vi "GTRC HPOC UI.vi"() -> ()   [LabVIEW 2018]
uses:
  <vilib>/DAQmx/read.llb/DAQmx Read (Analog 1D DBL NChan 1Samp).vi
  <extravilib>/ChannelInstances/Lossy Stream-c(a[.](c(dbl,dbl,dbl,dbl)),stamp,a[.](dbl),c(dbl,dbl,dbl,dbl,dbl,dbl,dbl))/Read With Abort.vi
  <extravilib>/ChannelInstances/High Speed Stream-c(a[.](c(dbl,dbl,dbl,dbl)),stamp,a[.](dbl),c(dbl,dbl,dbl,dbl,dbl,dbl,dbl))/_Read For Replicate.vi
  <extravilib>/ChannelInstances/Lossy Stream-c(a[.](c(dbl,dbl,dbl,dbl)),stamp,a[.](dbl),c(dbl,dbl,dbl,dbl,dbl,dbl,dbl))/Write With Abort.vi
  <extravilib>/ChannelInstances/Lossy Stream-c(a[.](c(dbl,dbl,dbl,dbl)),stamp,a[.](dbl),c(dbl,dbl,dbl,dbl,dbl,dbl,dbl))/EndpointRead.vi
  <extravilib>/ChannelInstances/Lossy Stream-c(a[.](c(dbl,dbl,dbl,dbl)),stamp,a[.](dbl),c(dbl,dbl,dbl,dbl,dbl,dbl,dbl))/Endpoint.vi
  <extravilib>/ChannelInstances/Lossy Stream-c(a[.](c(dbl,dbl,dbl,dbl)),stamp,a[.](dbl),c(dbl,dbl,dbl,dbl,dbl,dbl,dbl))/Instantiate.vi
  <extravilib>/ChannelInstances/Lossy Stream-c(a[.](c(dbl,dbl,dbl,dbl)),stamp,a[.](dbl),c(dbl,dbl,dbl,dbl,dbl,dbl,dbl))/)Channel.vi
  <resource>/ChannelSupport/_ChannelSupport/WaitIfNeeded.vi
  <extravilib>/ChannelInstances/High Speed Stream-c(a[.](c(dbl,dbl,dbl,dbl)),stamp,a[.](dbl),c(dbl,dbl,dbl,dbl,dbl,dbl,dbl))/Instantiate.vi
  <extravilib>/ChannelInstances/High Speed Stream-c(a[.](c(dbl,dbl,dbl,dbl)),stamp,a[.](dbl),c(dbl,dbl,dbl,dbl,dbl,dbl,dbl))/)Channel.vi
  <extravilib>/ChannelInstances/High Speed Stream-c(a[.](c(dbl,dbl,dbl,dbl)),stamp,a[.](dbl),c(dbl,dbl,dbl,dbl,dbl,dbl,dbl))/Abort Signal/Init Signal.vi
  <vilib>/Utility/file.llb/Write Delimited Spreadsheet (string).vi
  <vilib>/DAQmx/create/channels.llb/DAQmx Create Channel (AI-Temperature-Thermocouple).vi
  <vilib>/DAQmx/configure/timing.llb/DAQmx Timing (Sample Clock).vi
  <vilib>/DAQmx/miscellaneous.llb/DAQmx Fill In Error Info.vi
  <extravilib>/ChannelInstances/High Speed Stream-c(a[.](c(dbl,dbl,dbl,dbl)),stamp,a[.](dbl),c(dbl,dbl,dbl,dbl,dbl,dbl,dbl)).lvlib
  <resource>/objmgr/daqmx.rc
  <extravilib>/ChannelInstances/Lossy Stream-c(a[.](c(dbl,dbl,dbl,dbl)),stamp,a[.](dbl),c(dbl,dbl,dbl,dbl,dbl,dbl,dbl)).lvlib
panel:
  out "Driving Variables":T1
  in  "Line Controls\n(Don't Delete)":T2(tab)
  in  "Line Flowrate Control":T3 {"Line 5" scale=0.0..5.0; "Line 4" scale=0.0..4.0; "Line 3" scale=0.0..3.0; "Line 2" scale=0.0..8.0; "Line 1" scale=0.0..9.0}
  in  "Temperatures Control":T3 {"Line 5" scale=0.0..10.0; "Line 4" scale=0.0..10.0; "Line 3" scale=0.0..10.0; "Line 2" scale=0.0..10.0; "Line 1" scale=0.0..10.0}
  in  "Pressure Controls":T3 {"Line 5" scale=0.0..10.0; "Line 4" scale=0.0..10.0; "Line 3" scale=0.0..10.0; "Line 2" scale=0.0..10.0; "Line 1" scale=0.0..10.0}
  in  "Species List":string[][](table)=[["Custom", "9999999999", ""], ["Methanol", "6.47", "19.93"], ["Butanol", "11.2", "33.075"], ["Propane", "15.67", "46.35"], ["Methane", "13.19", "50.00"], ["Hydrogen", "34.3", "119.96"], ["Ammonia", "6.0466", "22.5"], ["Pentane", "15.32", "45.36"], ["Butane", "14.98", "45.75"], ["Hexane", "15.24", "44.75"], ["Ethanol", "9", "26.70"], ["Empty (Not Used)", "0", "0"]]
  in  "Rig Temperature Tab Box\n(Don't Delete)":enum32{"Rig Temps Live", "Alarm Thresholds"}(tab)
  out "Rig Temperatures":T4
  in  "Rig Alarm Thresholds":T4
  out "DAQ Current Time":timestamp format="%<%X>T"
  in  "UI Refresh Rate (Hz)":u32=1 min=1 max=500 step=1
  out "Line Pressures":T5(graph)
  out "Line Temperatures":T5(graph)
  in  "Lines Tab Control\n(Don't delete)":enum32{"Live Data", "AFR Info", "Setup Lines"}(tab)
  out "Flowrate Data":T6(array[cluster]) {"Line Number" format="%#.1g"; "Temperature" format="%.2g"; "Pressure" format="%.2g"; "Flowrate" format="%.2g"}
  out "AFR Display":T7(array[cluster])
  in  "Line Setup":T8(array[cluster])
  out "Actual Sample Rate":dbl
  out "Export Timestamp":timestamp format="%<%H:%M:%S>T"
  out "UI Timestamp":timestamp format="%<%X\n%x>T"
  in  "file path (dialog if empty)":path
  out "Export Loop Status":T9(ring)
  in  "Start Recording?":bool
  in  "Stop Recording?":bool
  out "Acquisition Loop Status":T10(ring)
  in  "Begin Acquisition":bool
  in  "DAQ Properties":cluster{"Sample Rate [Hz]":dbl}={"Sample Rate [Hz]"=1.0} {"Sample Rate [Hz]" min=1.0 max=5000.0 step=1.0}
  # "Loop Status"
  # "Rig Temperatures [ °C]"
  # "Rig Thresholds [ °C]"
  # "Live \n Live Line Data"
  # "°C"
  # "Bar"
  # "g/s"
  # "Air-to-Fuel Ratios for each Line"
  # "Line Setup"
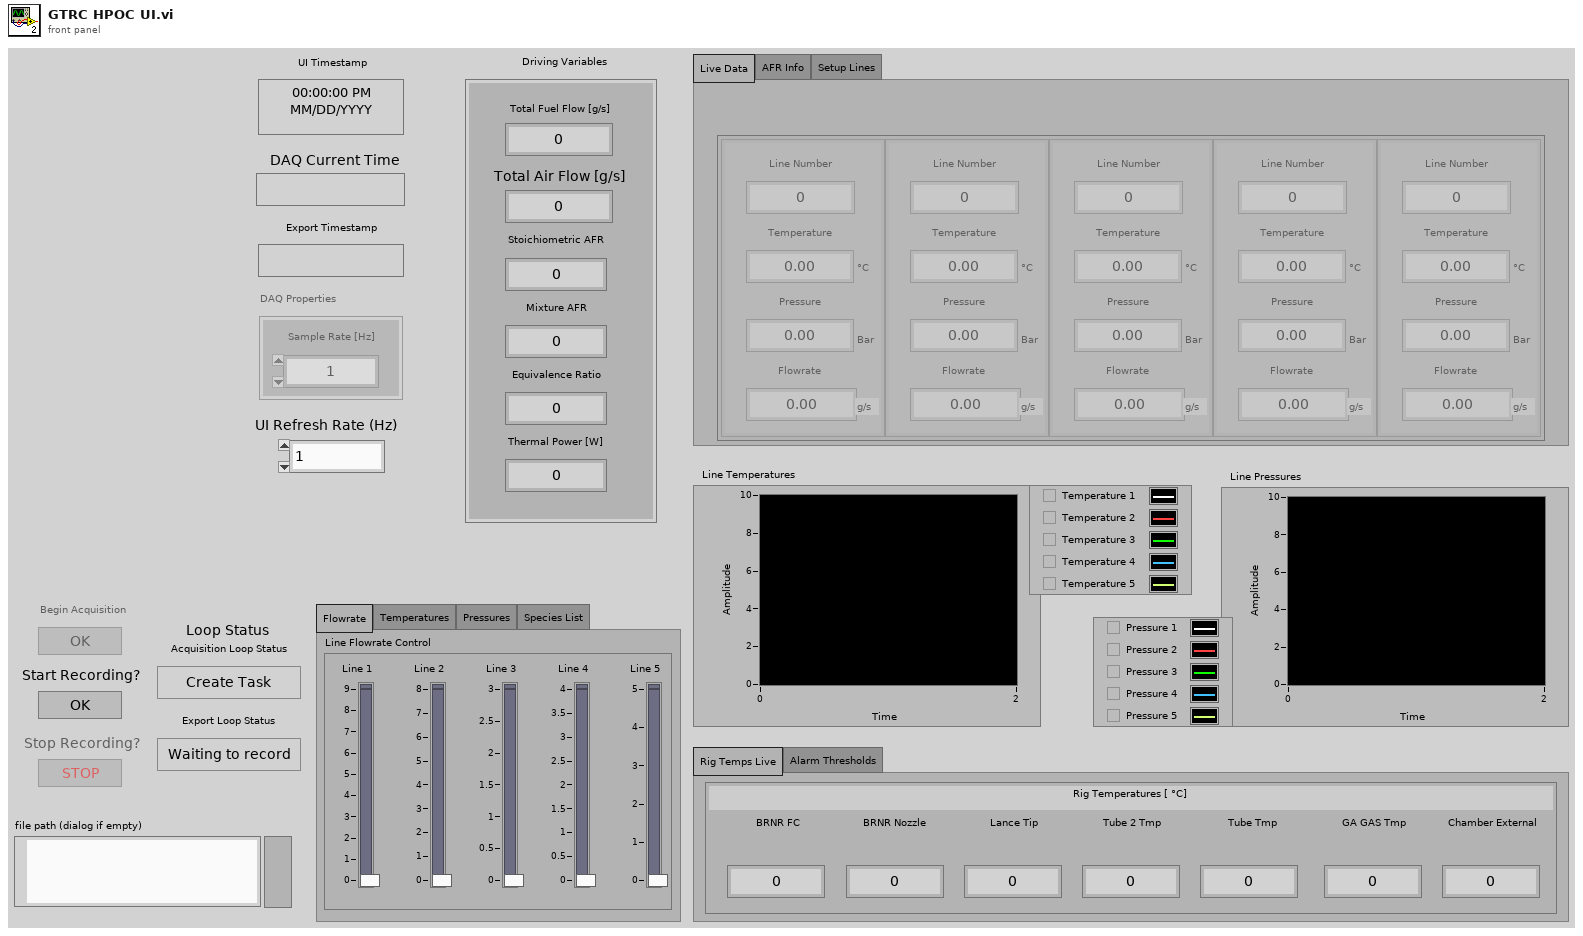
[diagram p1: front panel]
types:
  T1 = cluster{"Total Air Flow [g/s]":dbl, "Total Fuel Flow [g/s]":dbl, "Mixture AFR":dbl, "Stoichiometric AFR":dbl, "Equivalence Ratio":dbl, "Thermal Power [W]":dbl}
  T2 = enum32{"Flowrate", "Temperatures", "Pressures", "Species List"}
  T3 = cluster{"Line 1":dbl, "Line 2":dbl, "Line 3":dbl, "Line 4":dbl, "Line 5":dbl}
  T4 = cluster{"BRNR FC":dbl, "BRNR Nozzle":dbl, "Lance Tip":dbl, "Tube 2 Tmp":dbl, "Tube Tmp":dbl, "GA GAS Tmp":dbl, "Chamber External":dbl}
  T5 = cluster{"[0]":dbl, "[1]":dbl, "[2]":dbl, "[3]":dbl, "[4]":dbl}
  T6 = cluster{"Line Number":dbl, "Temperature":dbl, "Pressure":dbl, "Flowrate":dbl}[]
  T7 = cluster{"Line Number":i32, "AFR":dbl, "Species":enum16{"Empty (Not used)", "Custom", "Air", "Methanol", "Ethanol", "Butanol", "Propane", "Methane", "Hydrogen", "Pentane", "Butane", "Hexane"}}[]
  T8 = cluster{"Custom AFR":dbl, "Species":enum16{"Empty (Not used)", "Custom", "Air", "Methanol", "Ethanol", "Butanol", "Propane", "Methane", "Hydrogen", "Pentane", "Butane", "Hexane"}, "Custom Lower Heating Value [kJ/kg]":dbl}[]
  T9 = enum16{"Waiting to record", "Creating Spreadsheet", "Recording", "Finished Recording"}
  T10 = enum16{"Create Task", "Change Settings", "Check Settings", "Read Data", "End Task"}
  T11 = enum8{"Enabled", "Disabled", "Disabled and Grayed Out"}
  T12 = cluster{"Flowrate Data":cluster{"Line Number":dbl, "Temperature":dbl, "Pressure":dbl, "Flowrate":dbl}[], "Current Time":timestamp, "DAQmx Data":dbl[], "Rig Temperatures":cluster{"BRNR FC":dbl, "BRNR Nozzle":dbl, "Lance Tip":dbl, "Tube 2 Tmp":dbl, "Tube Tmp":dbl, "GA GAS Tmp":dbl, "Chamber External Temp":dbl}}
  T13 = cluster{"BRNR FC":dbl, "BRNR Nozzle":dbl, "Lance Tip":dbl, "Tube 2 Tmp":dbl, "Tube Tmp":dbl, "GA GAS Tmp":dbl, "Chamber External Temp":dbl}
  T14 = typedef "High Speed Stream-c(a[.](c(dbl,dbl,dbl,dbl)),stamp,a[.](dbl),c(dbl,dbl,dbl,dbl,dbl,dbl,dbl)).lvlib/)Channel.ctl" = refnum<queue>
  T15 = typedef "Lossy Stream-c(a[.](c(dbl,dbl,dbl,dbl)),stamp,a[.](dbl),c(dbl,dbl,dbl,dbl,dbl,dbl,dbl)).lvlib/)Channel.ctl" = refnum<queue>
  T16 = cluster{"Line":i32, "AFR":dbl, "Species":enum16{"Empty (Not used)", "Custom", "Air", "Methanol", "Ethanol", "Butanol", "Propane", "Methane", "Hydrogen", "Pentane", "Butane", "Hexane"}}
  T17 = enum16{"Empty (Not used)", "Custom", "Air", "Methanol", "Ethanol", "Butanol", "Propane", "Methane", "Hydrogen", "Pentane", "Butane", "Hexane"}
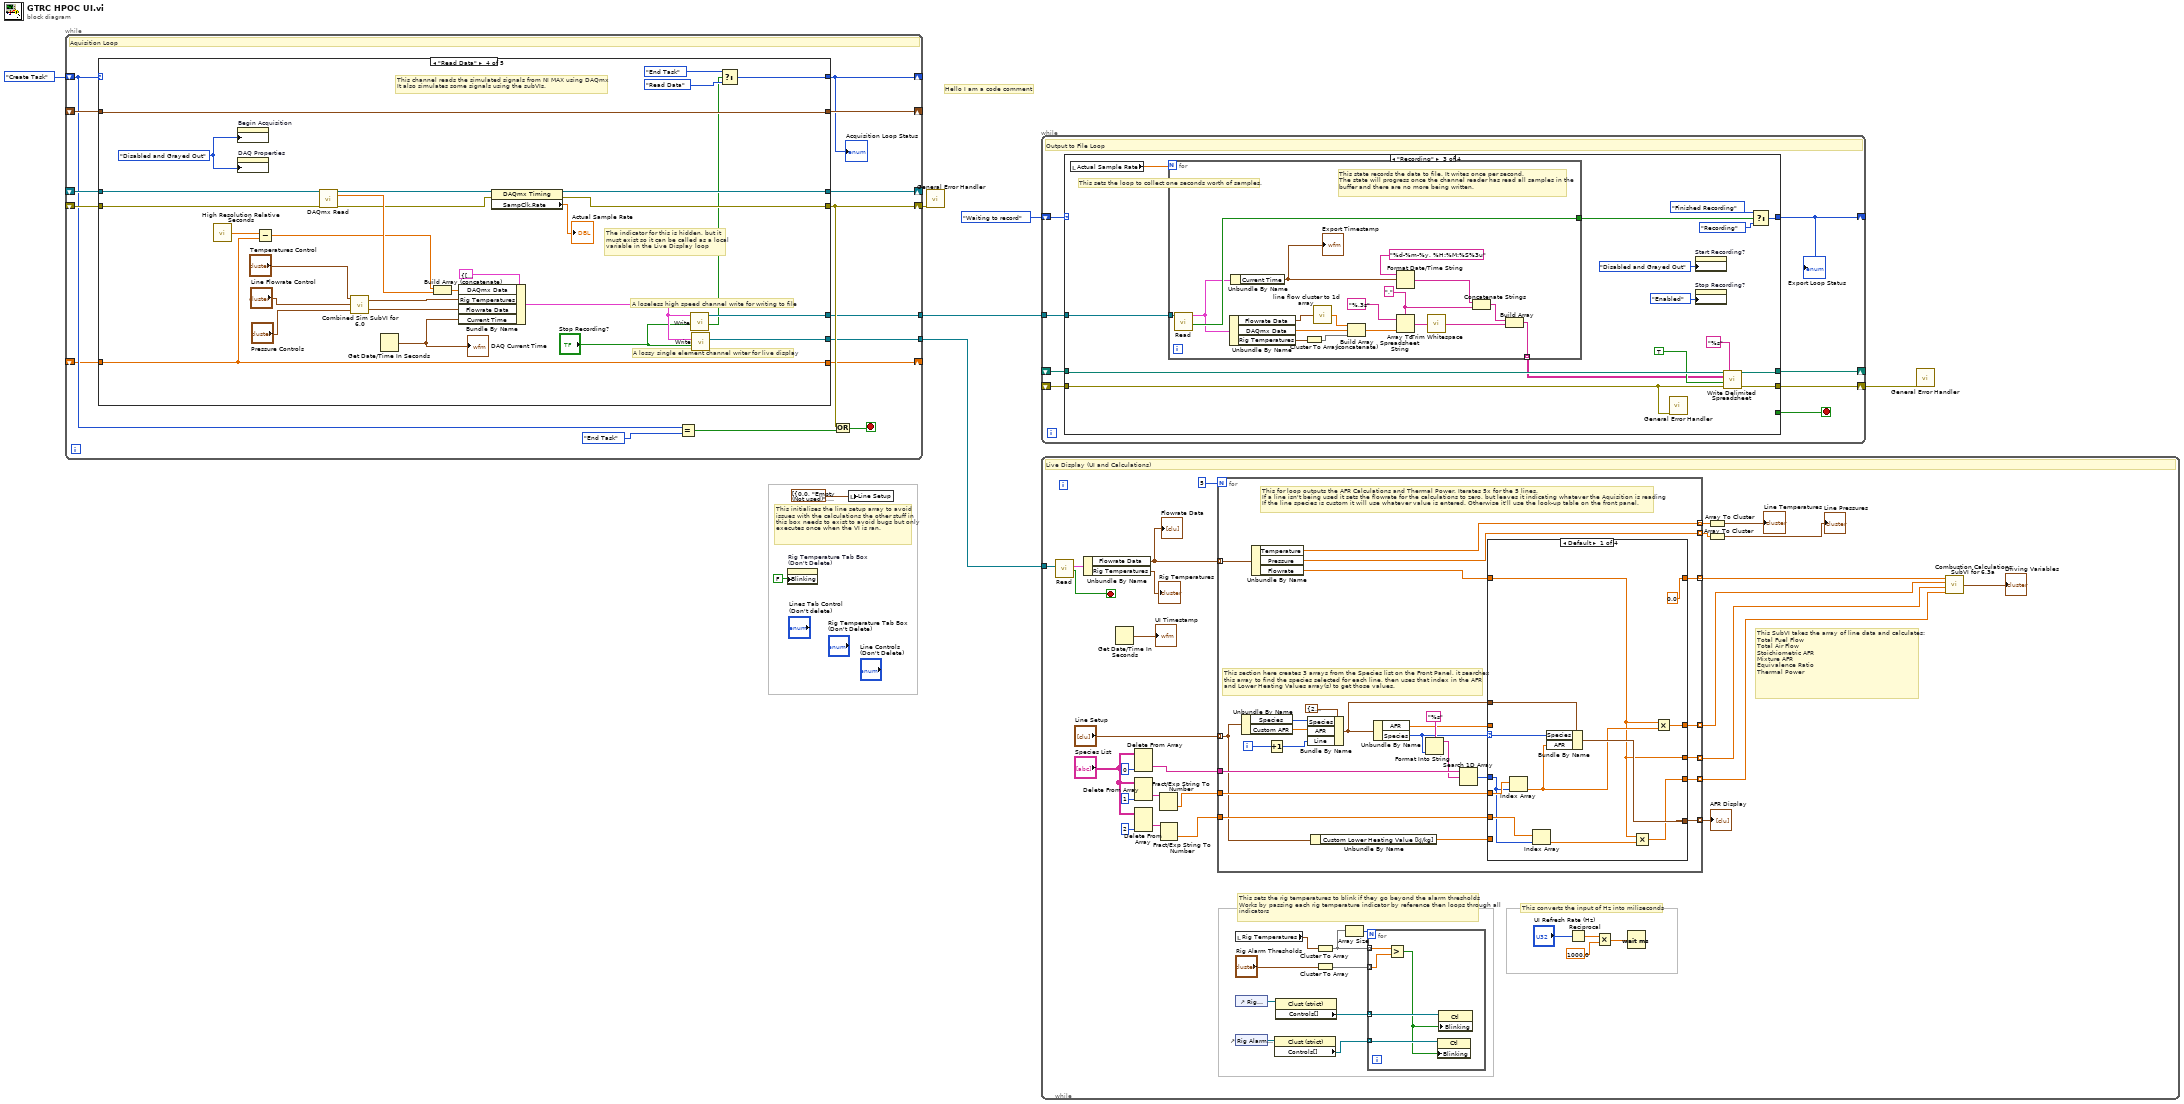
[diagram p0: block diagram]
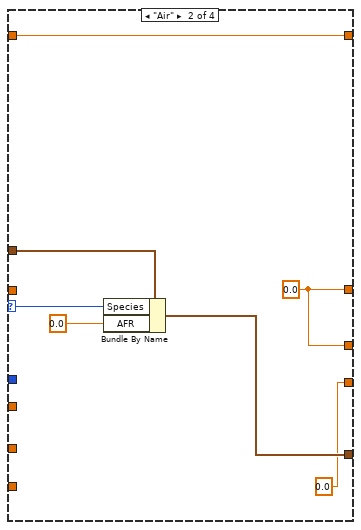
[diagram p2: hidden frame]
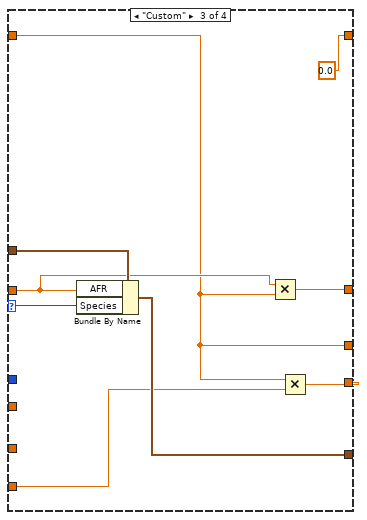
[diagram p3: hidden frame]
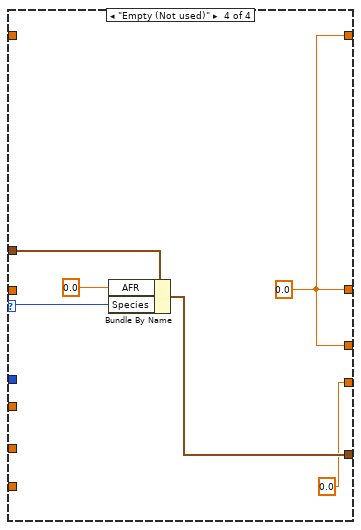
[diagram p4: hidden frame]
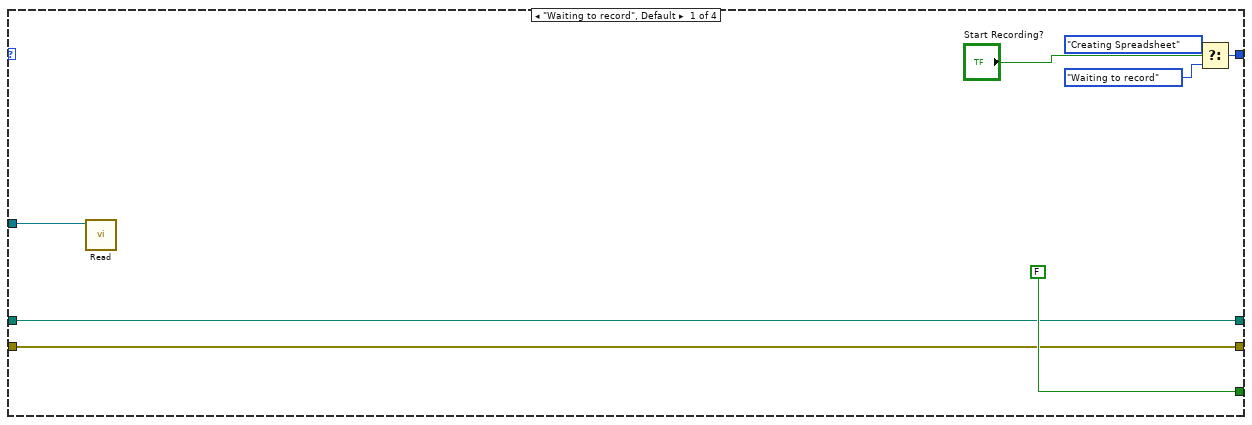
[diagram p5: hidden frame]
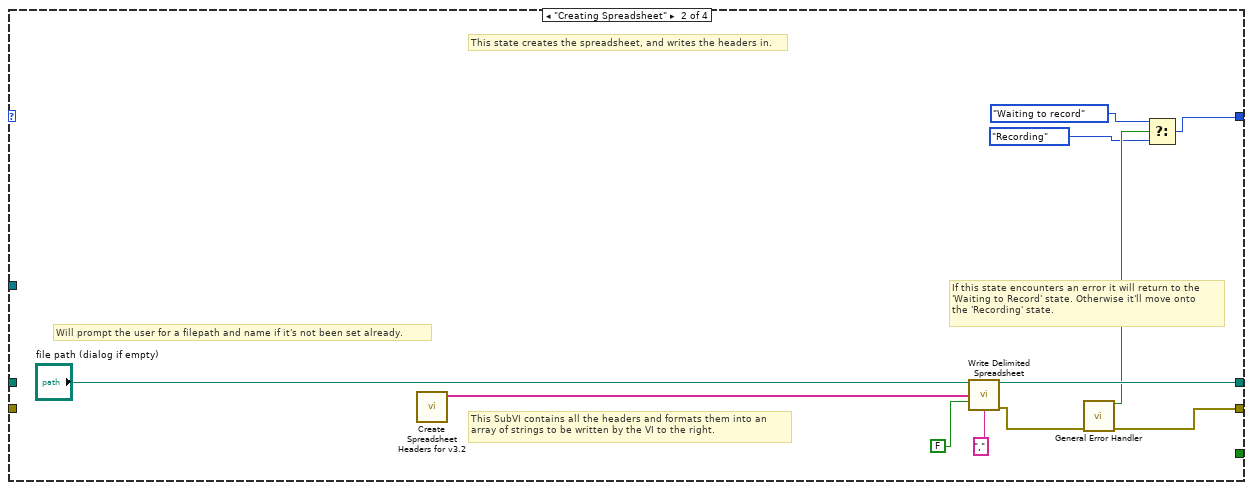
[diagram p6: hidden frame]
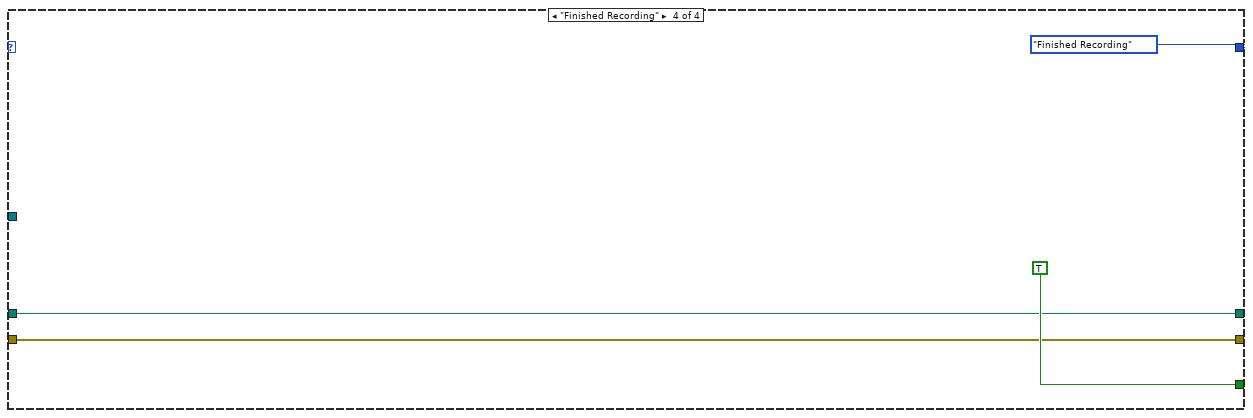
[diagram p7: hidden frame]
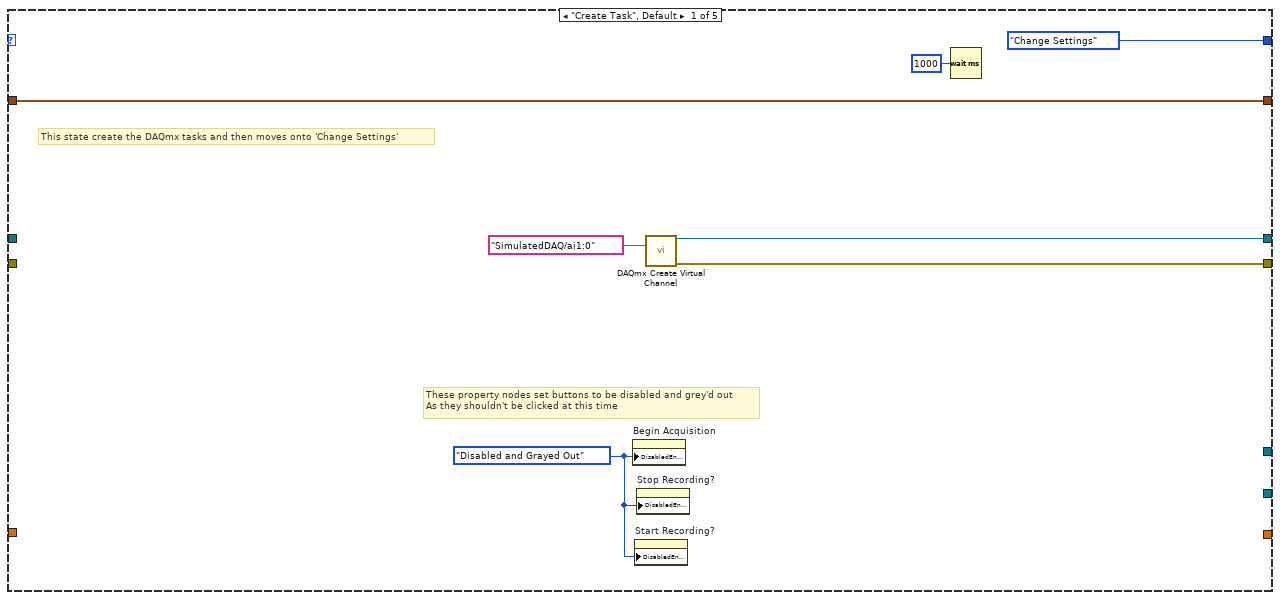
[diagram p8: hidden frame]
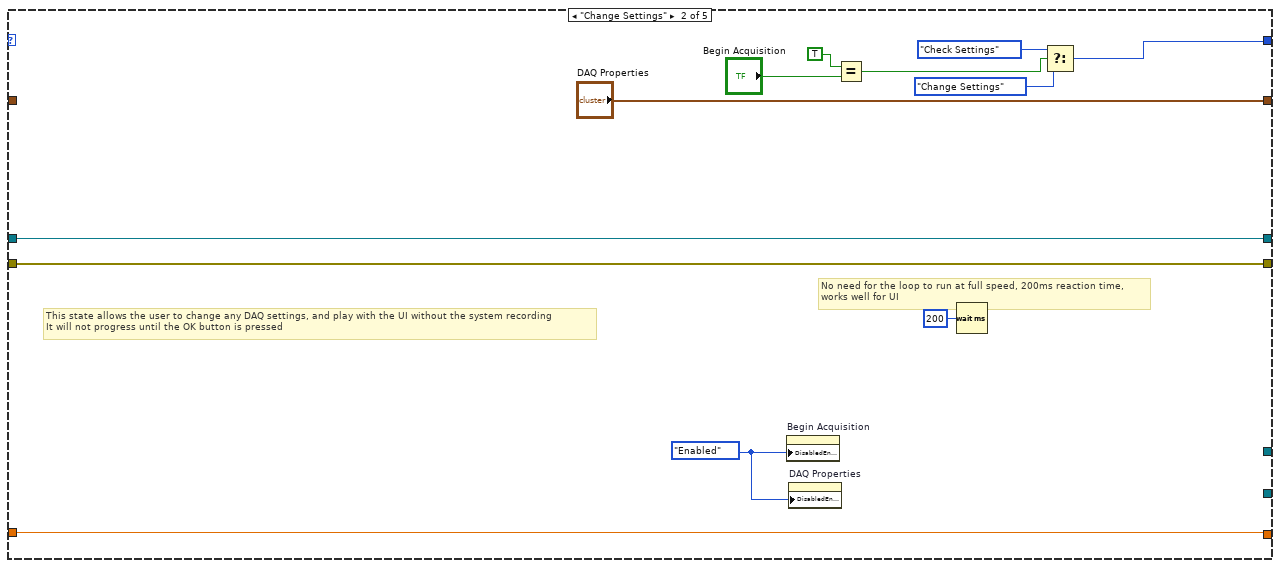
[diagram p9: hidden frame]
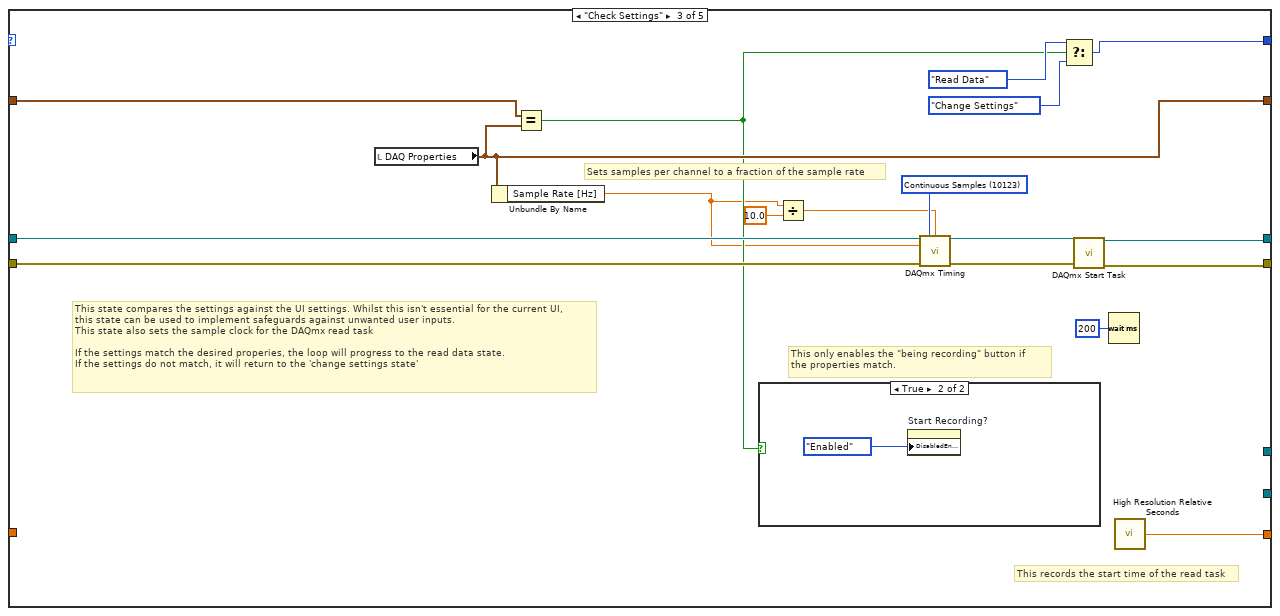
[diagram p10: hidden frame]
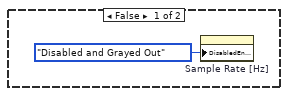
[diagram p11: hidden frame]
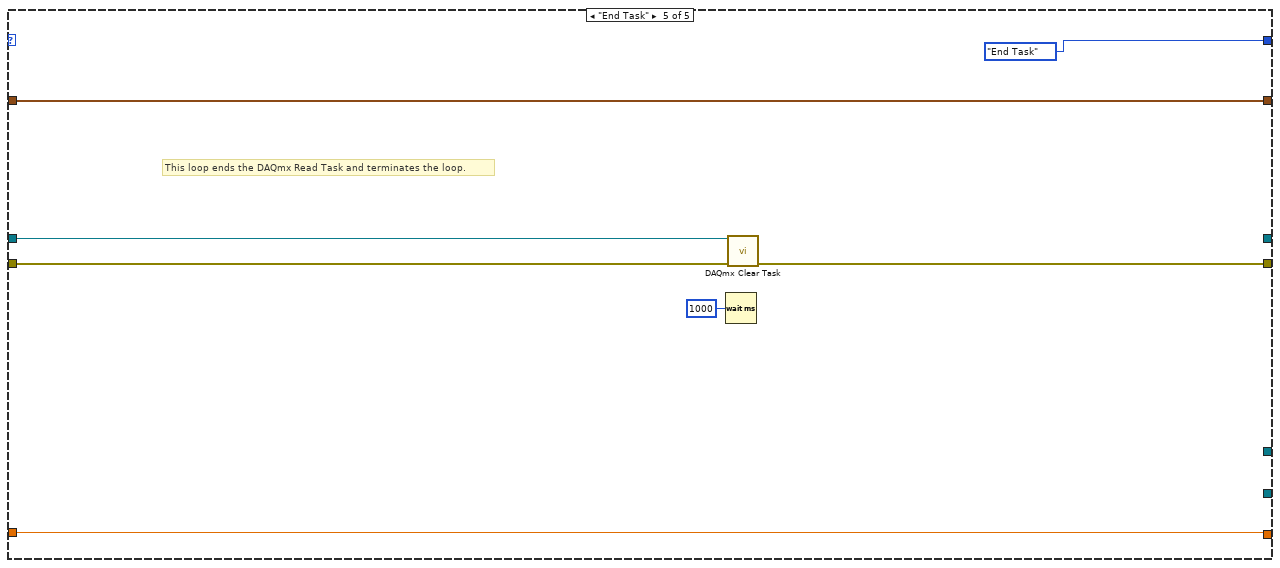
[diagram p12: hidden frame]
diagram:
  # "Hello I am a code comment"
  # "This initialises the line setup array to avoid issues with the calculations the other stuff in this box needs to exist to avoid bugs but only executes once when the VI is ran."
  n1 = while {
    shift-right: [w18] -> _
    shift-left: T10."Create Task" -> [w14]
    shift-right: [w23] -> _
    shift-left: _ -> [w21]
    shift-right: [w17] -> w4
    shift-left: _ -> [w20]
    shift-right: [w22] -> _
    shift-left: _ -> [w19]
    tunnel: [w13] -> w6
    tunnel: [w11] -> w3
    shift-right: [w9] -> _
    shift-left: _ -> [w10]
    stop <- w12 stop-if-true
    # "Aquisition Loop"
    n2 = case shown="\"Read Data\"" w14 {
      tunnel: [w30 w42 w50 w78 _] -> w23
      tunnel: [w29 w41 w49 w79 w98] -> w17
      tunnel: [T10."Change Settings" w35 w56 w87 T10."End Task"] -> w18
      tunnel: [w26 "DAQ Properties" w53 w89 w97] -> w22
      tunnel: w21 -> [_ w42 w55 w91 w95]
      tunnel: w20 -> [_ w41 w54 w90 w94]
      tunnel: w19 -> [w26 _ w60 w89 w97]
      tunnel: [_ _ _ w83 _] -> w13
      tunnel: [_ w31 w43 w74 w92] -> w9
      tunnel: w10 -> [_ w31 _ w74 w92]
      tunnel: [_ _ _ w71 _] -> w11
      frame "Create Task", Default {
        w24 = T11."Disabled and Grayed Out" ("Disabled")
        # "These property nodes set buttons to be disabled and grey'd out\nAs they shouldn't be clicked at this time"
        # "This state create the DAQmx tasks and then moves onto 'Change Settings'"
        n3 = property on="Begin Acquisition" class="Bool"("DisabledEnum"=w24) -> ()  [unwired: 2 in, 2 out]
        n4 = property on="Start Recording?" class="Bool"("DisabledEnum"=w24) -> ()  [unwired: 2 in, 2 out]
        n5 = property on="Stop Recording?" class="Bool"("DisabledEnum"=w24) -> ()  [unwired: 2 in, 2 out]
        n6 = call-poly <vilib>:"DAQmx Create Virtual Channel.vi"("physical channels"=tag "SimulatedDAQ/ai1:0") -> ("task out"=w30:refnum<k21>, "error out"=w29:errorcluster)  [unwired: 13 in]
        n7 = Wait (ms)(milliseconds to wait=u32 1000) -> ()  [unwired: 1 out]
      }
      frame "Change Settings" {
        w32 = T11."Enabled" ("Disabled")
        # "No need for the loop to run at full speed, 200ms reaction time,\nworks well for UI"
        # "This state allows the user to change any DAQ settings, and play with the UI without the system recording\nIt will not progress until the OK button is pressed"
        n8 = property on="Begin Acquisition" class="Bool"("DisabledEnum"=w32) -> ()  [unwired: 2 in, 2 out]
        n9 = property on="DAQ Properties" class="Clust (strict)"("DisabledEnum"=w32) -> ()  [unwired: 2 in, 2 out]
        n10 = Equal?(x=TRUE, y="Begin Acquisition") -> (x = y?=w37:bool)
        n11 = Wait (ms)(milliseconds to wait=u32 200) -> ()  [unwired: 1 out]
        n12 = Select(t=T10."Check Settings", s=w37, f=T10."Change Settings") -> (s? t:f=w35:T10)
      }
      frame "Check Settings" {
        w48 = 10123 items=["Finite Samples"=10178, "Continuous Samples"=10123, "Hardware Timed Single Point"=12522] ("sample mode")
        # "This records the start time of the read task"
        # "This only enables the \"being recording\" button if \nthe properties match."
        # "Sets samples per channel to a fraction of the sample rate"
        # "This state compares the settings against the UI settings. Whilst this isn't essential for the current UI, \nthis state can be used to implement safeguards against unwanted user inputs.\nThis state also sets the sample clock for the DAQmx read task\n\nIf the settings match the desired properies, the loop will progress to the read data state.\nIf the settings do not match, it will return to the 'change settings state'"
        n13 = local read "DAQ Properties"() -> (w53:cluster{"Sample Rate [Hz]":dbl})
        n14 = Unbundle By Name(w53) -> ("Sample Rate [Hz]"=w45:dbl)
        n15 = Equal?(x=w60, y=w53) -> (x = y?=w47:bool)
        n16 = case shown="True" w47 {
          frame False {
            n17 = property on="Sample Rate [Hz]" class="DigNum (strict)"("DisabledEnum"=T11."Disabled and Grayed Out" ("Disabled")) -> ()  [unwired: 2 in, 2 out]
          }
          frame True {
            n18 = property on="Start Recording?" class="Bool"("DisabledEnum"=T11."Enabled" ("Disabled")) -> ()  [unwired: 2 in, 2 out]
          }
        }
        n19 = Divide(x=w45, y=10.0) -> (x/y=w44:dbl)
        n20 = call-poly <vilib>:"DAQmx Timing.vi"("task/channels in"=w55, "sample mode"=w48, "samples per channel"=w44, "rate"=w45, "error in"=w54) -> ("task out"=w52:refnum<k21>, "error out"=w51:errorcluster)  [unwired: 9 in]
        n21 = Select(t=T10."Read Data", s=w47, f=T10."Change Settings") -> (s? t:f=w56:T10)
        n22 = call <vilib>:"DAQmx Start Task.vi"("task/channels in"=w52, "error in"=w51) -> ("task out"=w50:refnum<k21>, "error out"=w49:errorcluster)  [unwired: 12 in]
        n23 = Wait (ms)(milliseconds to wait=u32 200) -> ()  [unwired: 1 out]
        n24 = call <vilib>:"High Resolution Relative Seconds.vi"() -> ("relative seconds"=w43:dbl)
      }
      frame "Read Data" {
        w82 = T11."Disabled and Grayed Out" ("Disabled")
        # "This channel reads the simulated signals from NI MAX using DAQmx\nIt also simulates some signals using the subVIs."
        # "A lossy single element channel writer for live display"
        # "A loseless high speed channel write for writing to file"
        # "The indicator for this is hidden, but it\nmust exist so it can be called as a local \nvariable in the Live Display loop"
        n25 = call <vilib>:"High Resolution Relative Seconds.vi"() -> ("relative seconds"=w76:dbl)
        n26 = property on="Begin Acquisition" class="Bool"("DisabledEnum"=w82) -> ()  [unwired: 2 in, 2 out]
        n27 = property on="DAQ Properties" class="Clust (strict)"("DisabledEnum"=w82) -> ()  [unwired: 2 in, 2 out]
        n28 = Subtract(x=w76, y=w74) -> (x-y=w75:dbl)
        n29 = call-poly <vilib>:"DAQmx Read.vi"("task/channels in"=w91, "error in"=w90) -> ("task out"=w80:refnum<k21>, "data"=w85:dbl[], "error out"=w77:errorcluster)  [unwired: 11 in]
        n30 = call "Combined Sim SubVI for 6.0.vi"("Pressure Controls"="Pressure Controls", "Line Flowrate Control"="Line Flowrate Control", "Temperatures Control"="Temperatures Control") -> ("Flow Data"=w66:T6, "Rig Temperatures"=w67:T13)
        n31 = Get Date/Time In Seconds() -> (seconds since 1Jan1904=w68:timestamp)
        "DAQ Current Time" <- w68
        n32 = Build Array (concatenate)(w75, w85) -> (w69:dbl[])
        n33 = Bundle By Name(cluster=T12 {"Flowrate Data"=[{"Line Number"=1.0, "Temperature"=17.480721541683437, "Pressure"=24.0, "Flowrate"=0.0}, {"Line Number"=2.0, "Temperature"=21.850901927104296, "Pressure"=30.0, "Flowrate"=0.0}, {"Line Number"=3.0, "Temperature"=26.221082312525155, "Pressure"=36.0, "Flowrate"=0.0}, {"Line Number"=4.0, "Temperature"=30.591262697946018, "Pressure"=42.00000000000001, "Flowrate"=0.0}, {"Line Number"=5.0, "Temperature"=34.96144308336687, "Pressure"=48.0, "Flowrate"=0.0}], "Current Time"=timestamp(0 s since 1904-01-01), "DAQmx Data"=[], "Rig Temperatures"={"BRNR FC"=0.0, "BRNR Nozzle"=0.0, "Lance Tip"=0.0, "Tube 2 Tmp"=0.0, "Tube Tmp"=0.0, "GA GAS Tmp"=0.0, "Chamber External Temp"=0.0}}, "DAQmx Data"=w69, "Rig Temperatures"=w67, "Flowrate Data"=w66, "Current Time"=w68) -> (w81:T12)
        n34 = property class="DAQmx Timing"(reference=w80, error in=w77) -> (reference out=w78:refnum<k21>, error out=w79:errorcluster, "SampClk.Rate"=→"Actual Sample Rate":dbl)
        n35 = call <extravilib>:"Write.vi"("last element? (F)"="Stop Recording?", "element"=w81) -> ("done?"=w70:bool, "channel"=w83:T14)  [unwired: 7 in, 1 out]
        n36 = call <extravilib>:"Write.vi"("last element? (F)"="Stop Recording?", "element"=w81) -> ("channel"=w71:T15)  [unwired: 7 in, 2 out]
        n37 = Select(t=T10."End Task", s=w70, f=T10."Read Data") -> (s? t:f=w87:T10)
      }
      frame "End Task" {
        # "This loop ends the DAQmx Read Task and terminates the loop."
        n38 = Wait (ms)(milliseconds to wait=u32 1000) -> ()  [unwired: 1 out]
        n39 = call <vilib>:"DAQmx Clear Task.vi"("task in"=w95, "error in"=w94) -> ("error out"=w98:errorcluster)  [unwired: 13 in]
      }
    }
    "Acquisition Loop Status" <- w18
    n40 = Equal?(x=w14, y=T10."End Task") -> (x = y?=w15:bool)
    n41 = Or(x=w17, y=w15) -> (x .or. y?=w12:bool)
  }
  n42 = property on="Rig Temperature Tab Box\n(Don't Delete)" class="TabCtl (strict)"("Blinking"=FALSE) -> ()  [unwired: 2 in, 2 out]
  n43 = local write "Line Setup"(T8 [{"Custom AFR"=0.0, "Species"=enum."Empty (Not used)", "Custom Lower Heating Value [kJ/kg]"=0.0}, {"Custom AFR"=0.0, "Species"=enum."Empty (Not used)", "Custom Lower Heating Value [kJ/kg]"=0.0}, {"Custom AFR"=0.0, "Species"=enum."Empty (Not used)", "Custom Lower Heating Value [kJ/kg]"=0.0}, {"Custom AFR"=0.0, "Species"=enum."Empty (Not used)", "Custom Lower Heating Value [kJ/kg]"=0.0}, {"Custom AFR"=0.0, "Species"=enum."Empty (Not used)", "Custom Lower Heating Value [kJ/kg]"=0.0}] ("Line Setup")) -> ()
  n44 = call <vilib>:"General Error Handler.vi"("error in (no error)"=w4) -> ()  [unwired: 10 in, 5 out]
  n45 = while {
    shift-right: [w106] -> _
    shift-left: T9."Waiting to record" -> [w105]
    tunnel: w6 -> [w103]
    shift-right: [w101] -> _
    shift-left: _ -> [w102]
    shift-right: [w100] -> w5
    shift-left: _ -> [w99]
    stop <- w104 stop-if-true
    # "Output to File Loop"
    n46 = case shown="\"Recording\"" w105 {
      tunnel: [w111 w117 w139 T9."Finished Recording"] -> w106
      tunnel: [FALSE _ _ TRUE] -> w104
      tunnel: w103 -> [w107 _ w136 _]
      tunnel: w102 -> [w109 _ w133 w160]
      tunnel: [w109 w125 w134 w160] -> w101
      tunnel: [w108 w119 w130 w159] -> w100
      tunnel: w99 -> [w108 _ w126 w159]
      frame "Waiting to record", Default {
        n47 = call <extravilib>:"Read.vi"("channel"=w107) -> ()  [unwired: 6 in, 5 out]
        n48 = Select(t=T9."Creating Spreadsheet", s="Start Recording?", f=T9."Waiting to record") -> (s? t:f=w111:T9)
      }
      frame "Creating Spreadsheet" {
        # "Will prompt the user for a filepath and name if it's not been set already."
        # "If this state encounters an error it will return to the\n'Waiting to Record' state. Otherwise it'll move onto \nthe 'Recording' state."
        # "This SubVI contains all the headers and formats them into an\narray of strings to be written by the VI to the right."
        # "This state creates the spreadsheet, and writes the headers in."
        n49 = call "Create Spreadsheet Headers for v3.2.vi"() -> ("Array"=w124:string[])  [unwired: 11 in]
        n50 = call-poly <vilib>:"Write Delimited Spreadsheet.vi"("file path (dialog if empty)"="file path (dialog if empty)", "1D data"=w124, "append to file? (new file:F)"=FALSE, "delimiter (\\t)"="," ("delimiter (\\t)")) -> ("new file path (Not A Path if cancelled)"=w125:path, "error out"=w120:errorcluster)  [unwired: 10 in]
        n51 = call <vilib>:"General Error Handler.vi"("error in (no error)"=w120) -> ("error?"=w118:bool, "error out"=w119:errorcluster)  [unwired: 10 in, 3 out]
        n52 = Select(t=T9."Waiting to record", s=w118, f=T9."Recording") -> (s? t:f=w117:T9)
      }
      frame "Recording" {
        # "This sets the loop to collect one seconds worth of samples."
        n53 = local read "Actual Sample Rate"() -> (w127:dbl)
        n54 = for {
          N: w127 -> [_]
          tunnel: w136 -> [w157]
          tunnel: [w156] -> w135
          tunnel: [w141] -> w128 mode=indexing
          w146 = "," ("delimiter (Tab)")
          # "This state records the data to file. It writes once per second.\nThe state will progress once the channel reader has read all samples in the \nbuffer and there are no more being written."
          n55 = call <extravilib>:"Read.vi"("channel"=w157) -> ("done?"=w156:bool, "element"=w154:T12)  [unwired: 6 in, 3 out]
          n56 = Unbundle By Name(w154) -> ("Flowrate Data"=w155:T6, "DAQmx Data"=w152:dbl[], "Rig Temperatures"=w158:T13)
          n57 = Unbundle By Name(w154) -> ("Current Time"=w147:timestamp)
          "Export Timestamp" <- w147
          n58 = Cluster To Array(cluster=w158) -> (array=w153:dbl[])
          n59 = call "line flow cluster to 1d array.vi"("Flowrate Data"=w155) -> ("Array"=w151:dbl[])
          n60 = Build Array (concatenate)(w151, w152, w153) -> (w144:dbl[])
          n61 = Format Date/Time String(time format string (%c)="%d-%m-%y, %H:%M:%S%3u", seconds (now)=w147) -> (date/time string=w145:string)  [unwired: 1 in]
          n62 = Array To Spreadsheet String(delimiter (Tab)=w146, array=w144, 3:"%.3s" ("format string")) -> (spreadsheet string=w150:string)
          n63 = call <vilib>:"Trim Whitespace.vi"("string"=w150) -> ("trimmed string"=w142:string)  [unwired: 1 in]
          n64 = Concatenate Strings(w145, w146) -> (w143:string)
          n65 = Build Array(w143, w142) -> (w141:string[])
        }
        n66 = call <vilib>:"General Error Handler.vi"("error in (no error)"=w126) -> ()  [unwired: 10 in, 5 out]
        n67 = property on="Start Recording?" class="Bool"("DisabledEnum"=T11."Disabled and Grayed Out" ("Disabled")) -> ()  [unwired: 2 in, 2 out]
        n68 = property on="Stop Recording?" class="Bool"("DisabledEnum"=T11."Enabled" ("Disabled")) -> ()  [unwired: 2 in, 2 out]
        n69 = call-poly <vilib>:"Write Delimited Spreadsheet.vi"("file path (dialog if empty)"=w133, "format (%s)"="%s", "2D data"=w128, "append to file? (new file:F)"=TRUE, "error in (no error)"=w126) -> ("new file path (Not A Path if cancelled)"=w134:path, "error out"=w130:errorcluster)  [unwired: 9 in]
        n70 = Select(t=T9."Finished Recording", s=w135, f=T9."Recording") -> (s? t:f=w139:T9)
      }
      frame "Finished Recording" {
      }
    }
    "Export Loop Status" <- w106
  }
  n71 = while {
    tunnel: w3 -> [w201]
    stop <- w198 stop-if-true
    # "This SubVI takes the array of line data and calculates:\nTotal Fuel Flow\nTotal Air Flow\nStoichiometric AFR\nMixture AFR\nEquivalence Ratio\nThermal Power"
    # "This converts the input of Hz into miliseconds"
    # "This sets the rig temperatures to blink if they go beyond the alarm thresholds\nWorks by passing each rig temperature indicator by reference then loops through all indicators"
    # "Live Display (UI and Calculations)"
    n72 = call <extravilib>:"Read.vi"("channel"=w201) -> ("last element?"=w198:bool, "element"=w200:T12)  [unwired: 5 in, 4 out]
    n73 = Unbundle By Name(w200) -> ("Flowrate Data"=w183:T6, "Rig Temperatures"=→"Rig Temperatures":T13)
    "Flowrate Data" <- w183
    n74 = Get Date/Time In Seconds() -> (seconds since 1Jan1904=→"UI Timestamp":timestamp)
    n75 = Delete From Array(array="Species List", index (col)=0) -> (deleted portion=w191:string[])  [unwired: 2 in, 1 out]
    n76 = Delete From Array(array="Species List", index (col)=1 ("disabled index (col)")) -> (deleted portion=w192:string[])  [unwired: 2 in, 1 out]
    n77 = Delete From Array(array="Species List", index (col)=2 ("disabled index (col)")) -> (deleted portion=w171:string[])  [unwired: 2 in, 1 out]
    n78 = Fract/Exp String To Number(string=w192) -> (number=w193:dbl[])  [unwired: 3 in, 1 out]
    n79 = Fract/Exp String To Number(string=w171) -> (number=w170:dbl[])  [unwired: 3 in, 1 out]
    n80 = for {
      N: 5 -> [_]
      tunnel: w191 -> [w231]
      tunnel: w193 -> [w228]
      tunnel: "Line Setup" -> [w212] mode=indexing
      tunnel: [w219] -> w195 mode=indexing
      tunnel: w183 -> [w215] mode=indexing
      tunnel: [w218] -> w187 mode=indexing
      tunnel: [w217] -> w185 mode=indexing
      tunnel: w170 -> [w214]
      tunnel: [w213] -> w164 mode=indexing
      tunnel: [w210] -> w166 mode=indexing
      tunnel: [w209] -> w165 mode=indexing
      tunnel: [w208] -> w167 mode=indexing
      i -> [w221]
      # "This for loop outputs the AFR Calculations and Thermal Power. Iterates 5x for the 5 lines.\nIf a line isn't being used it sets the flowrate for the calculations to zero, but leaves it indicating whatever the Aquisition is reading\nIf the line species is custom it will use whatever value is entered. Otherwise it'll use the look-up table on the front panel."
      # "This section here creates 3 arrays from the Species list on the Front Panel, it searches \nthis array to find the species selected for each line, then uses that index in the AFR \nand Lower Heating Values array(s) to get those values."
      n81 = Unbundle By Name(w212) -> ("Species"=w225:T17, "Custom AFR"=w224:dbl)
      n82 = Unbundle By Name(w215) -> ("Temperature"=w218:dbl, "Pressure"=w217:dbl, "Flowrate"=w216:dbl)
      n83 = Increment(x=w221) -> (x+1=w222:i32)
      n84 = Bundle By Name(cluster=T16 {"Line"=2, "AFR"=1.0, "Species"=enum."Butane"} ("AFR Inputs"), "Species"=w225, "AFR"=w224, "Line"=w222) -> (w220:T16)
      n85 = Unbundle By Name(w212) -> ("Custom Lower Heating Value [kJ/kg]"=w211:dbl)
      n86 = Unbundle By Name(w220) -> ("AFR"=w229:dbl, "Species"=w226:T17)
      n87 = Format Into String(format string="%s", w226) -> (resulting string=w230:string)  [unwired: 2 in, 1 out]
      n88 = Search 1D Array(1D array=w231, element=w230) -> (index of element=w227:i32)  [unwired: 1 in]
      n89 = case shown="Default" w226 {
        selector: w226 -> [w243 w251 w258 w264]
        tunnel: w229 -> [_ _ w255 _]
        tunnel: w228 -> [w244 _ _ _]
        tunnel: w227 -> [w239 _ _ _]
        tunnel: [w241 w250 w260 w266] -> w219
        tunnel: w220 -> [w242 w249 w259 w265]
        tunnel: w216 -> [w234 w245 w253 _]
        tunnel: w214 -> [w240 _ _ _]
        tunnel: [w237 0.0 w254 0.0] -> w213
        tunnel: w211 -> [_ _ w252 _]
        tunnel: [w235 w246 w256 w261] -> w210
        tunnel: [w234 w246 w253 w261] -> w209
        tunnel: [0.0 ("Flowrate") w245 0.0 ("Flowrate") w261] -> w208
        frame Default {
          n90 = Index Array(array=w244, index=w239) -> (element=w236:dbl)
          n91 = Index Array(array=w240, index=w239) -> (element=w238:dbl)
          n92 = Bundle By Name(cluster=w242, "Species"=w243, "AFR"=w236) -> (w241:T16)
          n93 = Multiply(x=w234, y=w238) -> (x*y=w237:dbl)
          n94 = Multiply(x=w234, y=w236) -> (x*y=w235:dbl)
        }
        frame "Air" {
          w246 = 0.0
          n95 = Bundle By Name(cluster=w249, "Species"=w251, "AFR"=0.0) -> (w250:T16)
        }
        frame "Custom" {
          n96 = Bundle By Name(cluster=w259, "AFR"=w255, "Species"=w258) -> (w260:T16)
          n97 = Multiply(x=w255, y=w253) -> (x*y=w256:dbl)
          n98 = Multiply(x=w253, y=w252) -> (x*y=w254:dbl)
        }
        frame "Empty (Not used)" {
          w261 = 0.0 ("AFR")
          n99 = Bundle By Name(cluster=w265, "AFR"=0.0, "Species"=w264) -> (w266:T16)
        }
      }
    }
    "AFR Display" <- w195
    n100 = local read "Rig Temperatures"() -> (w181:T4)
    n101 = control-ref of="Rig Temperatures"() -> (w177:refnum<vi>)
    n102 = control-ref of="Rig Alarm Thresholds"() -> (w175:refnum<vi>)
    n103 = property class="Clust (strict)"(reference=w175) -> ("Controls[]"=w174:refnum<vi>[])  [unwired: 1 in, 2 out]
    n104 = property class="Clust (strict)"(reference=w177) -> ("Controls[]"=w176:refnum<vi>[])  [unwired: 1 in, 2 out]
    n105 = Cluster To Array(cluster=w181) -> (array=w178:dbl[])
    n106 = Cluster To Array(cluster="Rig Alarm Thresholds") -> (array=w180:dbl[])
    n107 = Array Size(array=w178) -> (size(s)=w179:i32)
    n108 = for {
      N: w179 -> [_]
      tunnel: w180 -> [w206] mode=indexing
      tunnel: w178 -> [w207] mode=indexing
      tunnel: w176 -> [w204] mode=indexing
      tunnel: w174 -> [w205] mode=indexing
      n109 = Greater?(x=w207, y=w206) -> (0:w203:bool)
      n110 = property on="Property Node" class="Ctl"(reference=w205, "Blinking"=w203) -> ()  [unwired: 1 in, 2 out]
      n111 = property on="Property Node" class="Ctl"(reference=w204, "Blinking"=w203) -> ()  [unwired: 1 in, 2 out]
    }
    n112 = Reciprocal(x="UI Refresh Rate (Hz)") -> (1/x=w169:dbl)
    n113 = Multiply(x=w169, y=1000.0) -> (x*y=w196:dbl)
    n114 = Wait (ms)(milliseconds to wait=w196) -> ()  [unwired: 1 out]
    n115 = Array To Cluster(array=w185) -> (cluster=→"Line Pressures":T5)
    n116 = Array To Cluster(array=w187) -> (cluster=→"Line Temperatures":T5)
    n117 = call "Combustion Calculations SubVI for 6.3a.vi"("Array of Thermal Powers"=w164, "Array of Fuel Flowrate"=w165, "Array of (Fuel Flow * AFR)"=w166, "Array of Air Flowrates"=w167) -> ("Driving Variables 2"=→"Driving Variables":T1)
  }
  n118 = call <vilib>:"General Error Handler.vi"("error in (no error)"=w5) -> ()  [unwired: 10 in, 5 out]
